vi "WriteData.vi"(9 "Data 2":dbl[](array[numeric]), 10 "Data":dbl[](array[numeric]), 11 "output cluster in":T1) -> (0 "Error Out":errorcluster, 3 "output cluster out":T1)   [LabVIEW 2016]
doc: "Writes last data to file"
uses:
  EK-P4/EK-P4.lvclass
  <userlib>/_MGI/File/Spreadsheet/MGI Write Spreadsheet Behavior Enum.ctl
  LoopData.ctl
panel:
  out "x = y?":bool
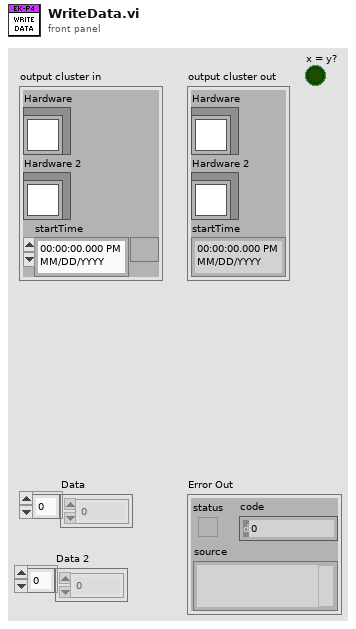
[diagram p1: front panel]
types:
  T1 = typedef "LoopData.ctl" = cluster{"Hardware":refnum<class "EK-P4.lvclass">, "Hardware 2":refnum<class "EK-P4.lvclass">, "startTime":timestamp}
  T2 = typedef "MGI Write Spreadsheet Behavior Enum.ctl" = enum16{"Append data", "Append headers and data", "Overwrite"}
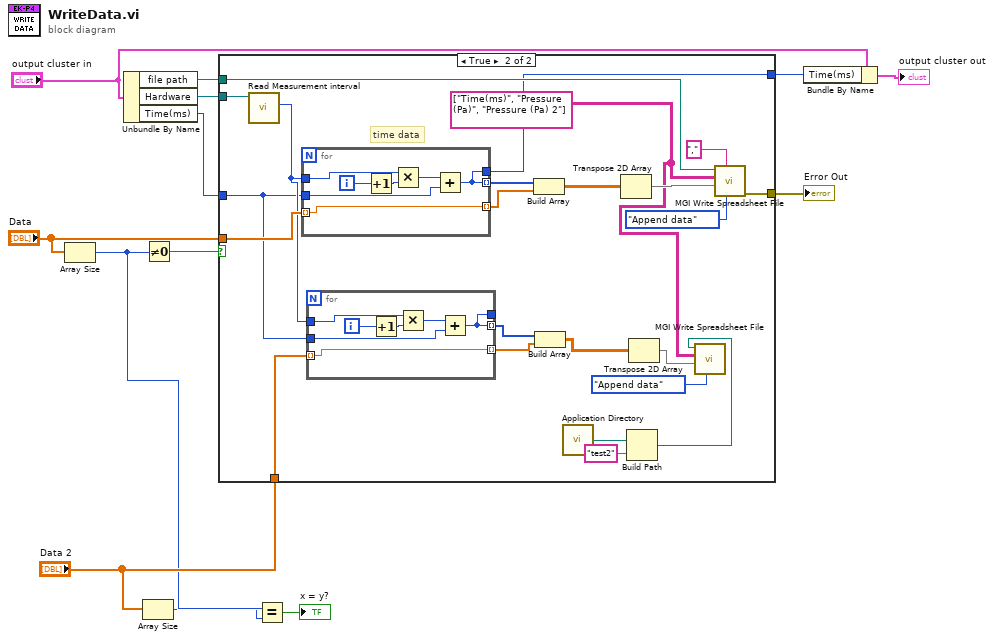
[diagram p0: block diagram]
diagram:
  n1 = Array Size(array="Data") -> (size(s)=w3:i32)
  n2 = Unbundle By Name("output cluster in") -> ("file path"=w10:path, "Hardware"=w11:refnum<class "EK-P4.lvclass">, "Time(ms)"=w5:i64)
  n3 = Array Size(array="Data 2") -> (size(s)=w2:i32)
  n4 = Not Equal To 0?(x=w3) -> (x != 0?=w6:bool)
  n5 = case shown="True" w6 {
    tunnel: w11 -> [_ w35]
    tunnel: w5 -> [w14 w24]
    tunnel: w10 -> [_ w34]
    tunnel: [w14 w33] -> w9
    tunnel: [_ w31] -> w8
    tunnel: "Data" -> [_ w28]
    tunnel: "Data 2" -> [_ w26]
    frame False {
    }
    frame True {
      w20 = string[][] [["Time(ms)", "Pressure (Pa)", "Pressure (Pa) 2"]] ("Header Lines[row][col]")
      # "time data"
      n6 = call-dynamic "Read Measurement interval.vi"("EK-P4 in"=w35) -> ("Measurement interval [ms]"=w25:u16)  [unwired: 8 in, 2 out]
      n7 = for {
        tunnel: w28 -> [w45] mode=indexing
        tunnel: w24 -> [w48]
        tunnel: w25 -> [w51]
        tunnel: [w47] -> w36 mode=indexing
        tunnel: [w47] -> w33
        tunnel: [w45] -> w27 mode=indexing
        i -> [w50]
        n8 = Increment(x=w50) -> (x+1=w46:i32)
        n9 = Multiply(x=w51, y=w46) -> (x*y=w49:i32)
        n10 = Add(x=w49, y=w48) -> (x+y=w47:i64)
      }
      n11 = for {
        tunnel: w26 -> [w38] mode=indexing
        tunnel: w24 -> [w41]
        tunnel: w25 -> [w44]
        tunnel: [w40] -> w23 mode=indexing
        tunnel: [w40] -> _
        tunnel: [w38] -> w22 mode=indexing
        i -> [w43]
        n12 = Increment(x=w43) -> (x+1=w39:i32)
        n13 = Multiply(x=w44, y=w39) -> (x*y=w42:i32)
        n14 = Add(x=w42, y=w41) -> (x+y=w40:i64)
      }
      n15 = Build Array(w36, w27) -> (w37:dbl[][])
      n16 = Build Array(w23, w22) -> (w21:dbl[][])
      n17 = call <vilib>:"Application Directory.vi"() -> ("Application Directory"=w17:path)
      n18 = Transpose 2D Array(2D array=w37) -> (transposed array=w29:dbl[][])
      n19 = Build Path(base path=w17, name or relative path="test2") -> (appended path=w15:path)
      n20 = Transpose 2D Array(2D array=w21) -> (transposed array=w19:dbl[][])
      n21 = call <userlib>:"MGI Write Spreadsheet File.vi"("Existing File Behavior"=MGI_Write_Spreadsheet_Behavior_Enum."Append data", "Data[row][col]"=w19, "Header Lines[row][col]"=w20, "Path"=w15) -> ()  [unwired: 4 in, 4 out]
      n22 = call <userlib>:"MGI Write Spreadsheet File.vi"("Existing File Behavior"=MGI_Write_Spreadsheet_Behavior_Enum."Append data", "Delimiter (Tab)"=",", "Data[row][col]"=w29, "Header Lines[row][col]"=w20, "Path"=w34) -> ("Error Out"=w31:errorcluster)  [unwired: 3 in, 3 out]
    }
  }
  "Error Out" <- w8
  n23 = Equal?(x=w3, y=w2) -> (x = y?=→"x = y?":bool)
  n24 = Bundle By Name(cluster="output cluster in", "Time(ms)"=w9) -> (→"output cluster out":T1)
